vi "Get LVObject.vi"(8 "error in (no error)":errorcluster, 11 "LVObjectMsg in":refnum<class "LVObjectMsg.lvclass">) -> (0 "error out":errorcluster, 2 "Message Data":refnum<class>, 3 "LVObjectMsg out":refnum<class "LVObjectMsg.lvclass">)   [LabVIEW 2013, in "LapDog.Messaging.v3.NativeTypes.lvlib" / "LVObjectMsg.lvclass"]
doc: "Returns the data contained in the message.\n\nThis method executes regardless of the error in state."
uses:
  LVObjectMsg.lvclass
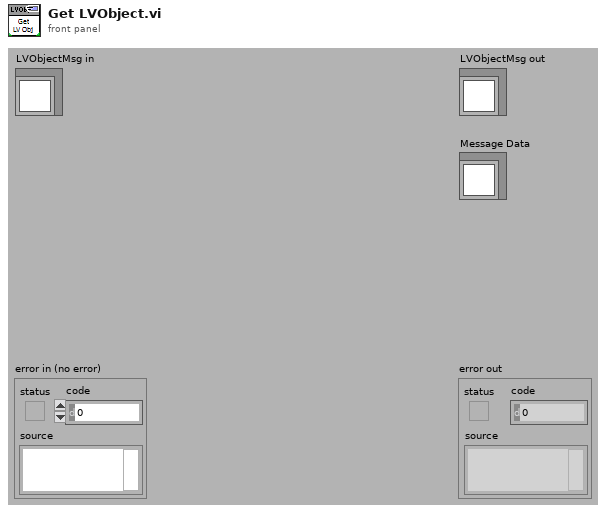
[diagram p1: front panel]
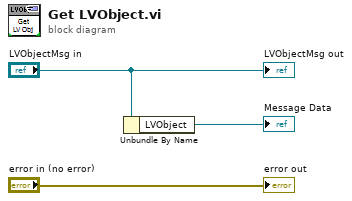
[diagram p0: block diagram]
diagram:
  n1 = Unbundle By Name("LVObjectMsg in") -> ("LVObject"=→"Message Data":refnum<class>)
  "error out" <- "error in (no error)"
  "LVObjectMsg out" <- "LVObjectMsg in"
